vi "Configure Range (Voltage).vi"(0 "VISA resource name":refnum<visa-resource-name>, 1 "Auto Range (F: Disable)":bool, 2 "Element (0:All)":i32(ring) items=["All", "1", "2", "3", "4", "5", "6"], 5 "Range Configuration (True)":bool[](array[boolean])=[TRUE, TRUE, TRUE, TRUE, TRUE, TRUE, TRUE, TRUE, TRUE, TRUE, TRUE, TRUE], 7 "Enable Peak Over Jump (F: Disable)":bool, 9 "Jump Range (1000 <500> V)":dbl(ring)=500.0 items=["1.5 <0.75>"=0.75, "3 <1.5>"=1.5, "6 <3>"=3.0, "10 <5>"=5.0, "15 <7.5>"=7.5, "30 <15>"=15.0, "60 <30>"=30.0, "100 <50>"=50.0, "150 <75>"=75.0, "300 <150>"=150.0, "600 <300>"=300.0, "1000 <500>"=500.0], 11 "error in (no error)":errorcluster, 12 "Manual Range (1000 <500> V)":dbl(ring)=500.0 items=["1.5 <0.75>"=0.75, "3 <1.5>"=1.5, "6 <3>"=3.0, "10 <5>"=5.0, "15 <7.5>"=7.5, "30 <15>"=15.0, "60 <30>"=30.0, "100 <50>"=50.0, "150 <75>"=75.0, "300 <150>"=150.0, "600 <300>"=300.0, "1000 <500>"=500.0]) -> (4 "VISA resource name out":refnum<visa-resource-name>, 15 "error out":errorcluster)   [LabVIEW 2021, in "Yokogawa WT1800 Series.lvlib"]
doc: "Configures the voltage range features."
uses:
  <instrlib>/Yokogawa WT1800 Series/Yokogawa WT1800 Series.lvlib
panel:
  # "1.5 <0.75> V"
  # "3 <1.5> V"
  # "6 <3> V"
  # "10 <5> V"
  # "15 <7.5> V"
  # "30 <15> V"
  # "60 <30> V"
  # "100 <50> V"
  # "150 <75> V"
  # "300 <150> V"
  # "600 <300> V"
  # "1000 <500> V"
  # "V"
  # "V"
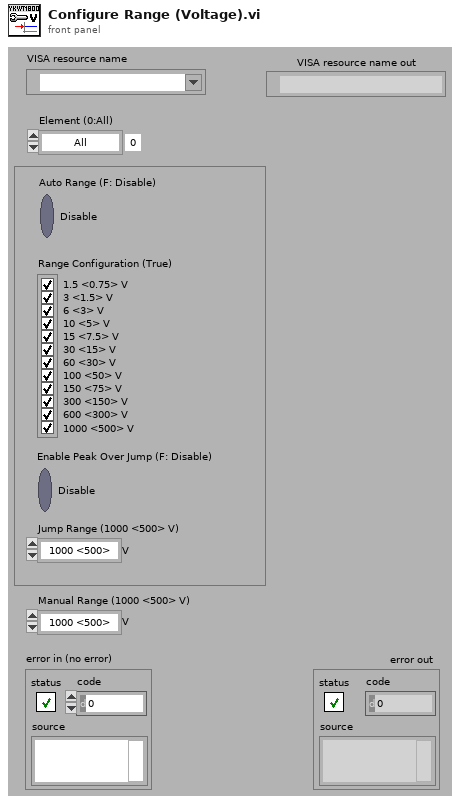
[diagram p1: front panel]
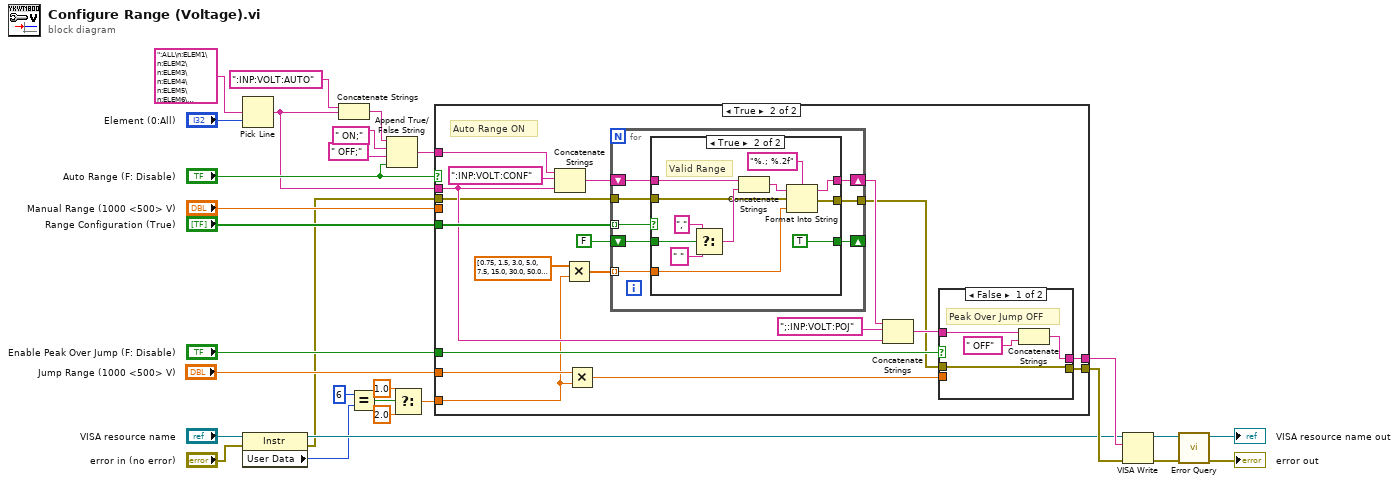
[diagram p0: block diagram]
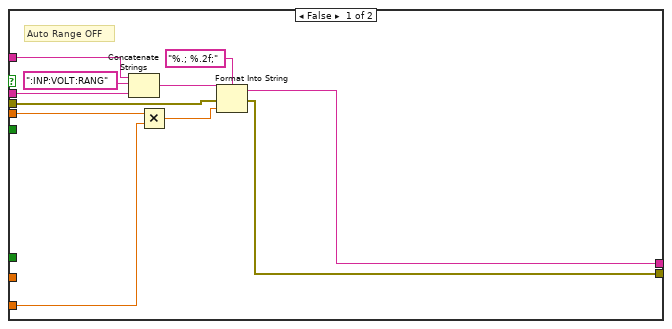
[diagram p2: hidden frame]
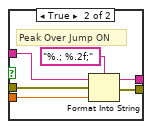
[diagram p3: hidden frame]
diagram:
  n1 = Pick Line ("ライン選択")(multi-line string=":ALL\n:ELEM1\n:ELEM2\n:ELEM3\n:ELEM4\n:ELEM5\n:ELEM6\n:SIGMA\n:SIGMB\n:SIGMC" ("複数行文字列"), line index="Element (0:All)") -> (output string=w18:string)  [unwired: 1 in]
  n2 = property class="Instr"(reference="VISA resource name", error in="error in (no error)") -> (reference out=w3:refnum<visa-resource-name>, error out=w2:errorcluster, "User Data"=w1:u32)
  n3 = Concatenate Strings(":INP:VOLT:AUTO", w18) -> (w20:string)
  n4 = Equal?(x=i64 6 ("y"), y=w1) -> (x = y?=w14:bool)
  n5 = Append True/False String ("True/False 文字列を追加")(1:"Auto Range (F: Disable)", 2:" OFF;", 3:" ON;", 4:w20) -> (0:w10:string)
  n6 = Select(t=1.0 ("y"), s=w14, f=2.0 ("y")) -> (s? t:f=w12:dbl)
  n7 = case shown="True" "Auto Range (F: Disable)" {
    tunnel: w18 -> [w35 w52]
    tunnel: "Manual Range (1000 <500> V)" -> [w37 _]
    tunnel: w12 -> [w36 w45]
    tunnel: "Range Configuration (True)" -> [_ w59]
    tunnel: w10 -> [w33 w56]
    tunnel: "Enable Peak Over Jump (F: Disable)" -> [_ w50]
    tunnel: "Jump Range (1000 <500> V)" -> [_ w46]
    tunnel: [w32 w48] -> w7
    tunnel: w2 -> [w31 w44]
    tunnel: [w30 w43] -> w6
    frame False {
      # "Auto Range OFF"
      n8 = Concatenate Strings(w33, ":INP:VOLT:RANG", w35) -> (w40:string)
      n9 = Multiply(x=w37, y=w36) -> (x*y=w38:dbl)
      n10 = Format Into String(format string="%.; %.2f;" ("形式文字列"), initial string=w40, error in=w31, w38) -> (resulting string=w32:string, error out=w30:errorcluster)
    }
    frame True {
      # "Auto Range ON"
      n11 = Concatenate Strings(w56, ":INP:VOLT:CONF", w52) -> (w58:string)
      n12 = Multiply(x=dbl[] [0.75, 1.5, 3.0, 5.0, 7.5, 15.0, 30.0, 50.0, 75.0, 150.0, 300.0, 500.0], y=w45) -> (x*y=w54:dbl[])
      n13 = Multiply(x=w46, y=w45) -> (x*y=w47:dbl)
      n14 = for {
        tunnel: w59 -> [w75] mode=indexing
        shift-right: [w76] -> w51
        shift-left: w58 -> [w77]
        tunnel: w54 -> [w74] mode=indexing
        tunnel: w44 -> [w73]
        tunnel: [w72] -> w42
        shift-right: [w70] -> _
        shift-left: FALSE -> [w71]
        n15 = case shown="True" w75 {
          tunnel: w77 -> [w80 w90]
          tunnel: [w80 w86] -> w76
          tunnel: w74 -> [_ w85]
          tunnel: w73 -> [w79 w84]
          tunnel: [w79 w83] -> w72
          tunnel: w71 -> [w78 w82]
          tunnel: [w78 TRUE] -> w70
          frame False {
            # "Invalid Range"
          }
          frame True {
            # "Valid Range"
            n16 = Select(t=",", s=w82, f=" ") -> (s? t:f=w89:string)
            n17 = Concatenate Strings(w90, w89) -> (w88:string)
            n18 = Format Into String(format string="%.; %.2f" ("形式文字列"), initial string=w88, error in=w84, w85) -> (resulting string=w86:string, error out=w83:errorcluster)
          }
        }
      }
      n19 = Concatenate Strings(w51, ";:INP:VOLT:POJ", w52) -> (w49:string)
      n20 = case shown="False" w50 {
        tunnel: w49 -> [w62 w68]
        tunnel: w47 -> [_ w67]
        tunnel: [w61 w66] -> w48
        tunnel: [w60 w65] -> w43
        tunnel: w42 -> [w60 w64]
        frame False {
          # "Peak Over Jump OFF"
          n21 = Concatenate Strings(w62, " OFF" ("文字列")) -> (w61:string)
        }
        frame True {
          # "Peak Over Jump ON"
          n22 = Format Into String(format string="%.; %.2f;" ("形式文字列"), initial string=w68, error in=w64, w67) -> (resulting string=w66:string, error out=w65:errorcluster)
        }
      }
    }
  }
  n23 = VISA Write ("VISA書き込み")(VISA resource name=w3, write buffer=w7, error in (no error)=w6) -> (VISA resource name out=w29:refnum<visa-resource-name>, error out=w28:errorcluster)  [unwired: 1 out]
  n24 = call <instrlib>:"Error Query.vi"("error in (no error)"=w28, "VISA resource name"=w29) -> ("error out"=→"error out":errorcluster, "VISA resource name out"=→"VISA resource name out":refnum<visa-resource-name>)  [unwired: 6 in, 2 out]
